vi "Store Reference.vi"(8 "error in":errorcluster, 11 "Reference":variant) -> (0 "error out":errorcluster, 3 "id":string)   [LabVIEW 2020, in "G-AI Core.lvlib"]
doc: "Stores a reference (e.g. VI Reference, Control Reference ...) in the G-AI Core and returns a unique id for later use of that reference.\n\n_____\nCreated using DQMH Framework: Event Scripter 7.1.2.1547."
uses:
  G-AI Core.lvlib
  Store Reference Argument--cluster.ctl
  Store Reference (Reply Payload)--cluster.ctl
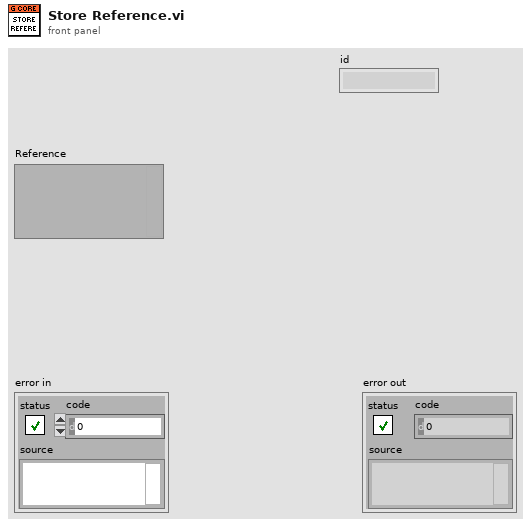
[diagram p1: front panel]
types:
  T1 = typedef "G-AI Core.lvlib/Store Reference Argument--cluster.ctl" = cluster{"Reference":variant, "Wait Notifier":refnum<notifier>, "wait for reply":bool}
  T2 = typedef "G-AI Core.lvlib/Request Events--cluster.ctl" = cluster{"Stop Module":refnum<user-event>, "Show Panel":refnum<user-event>, "Hide Panel":refnum<user-event>, "Get Module Execution Status":refnum<user-event>, "Show Diagram":refnum<user-event>, "Store Reference":refnum<user-event>, "Get Reference":refnum<user-event>, "New VI":refnum<user-event>, "Open VI Reference":refnum<user-event>}
  T3 = typedef "G-AI Core.lvlib/Store Reference (Reply Payload)--cluster.ctl" = cluster{"id":string, "error":errorcluster}
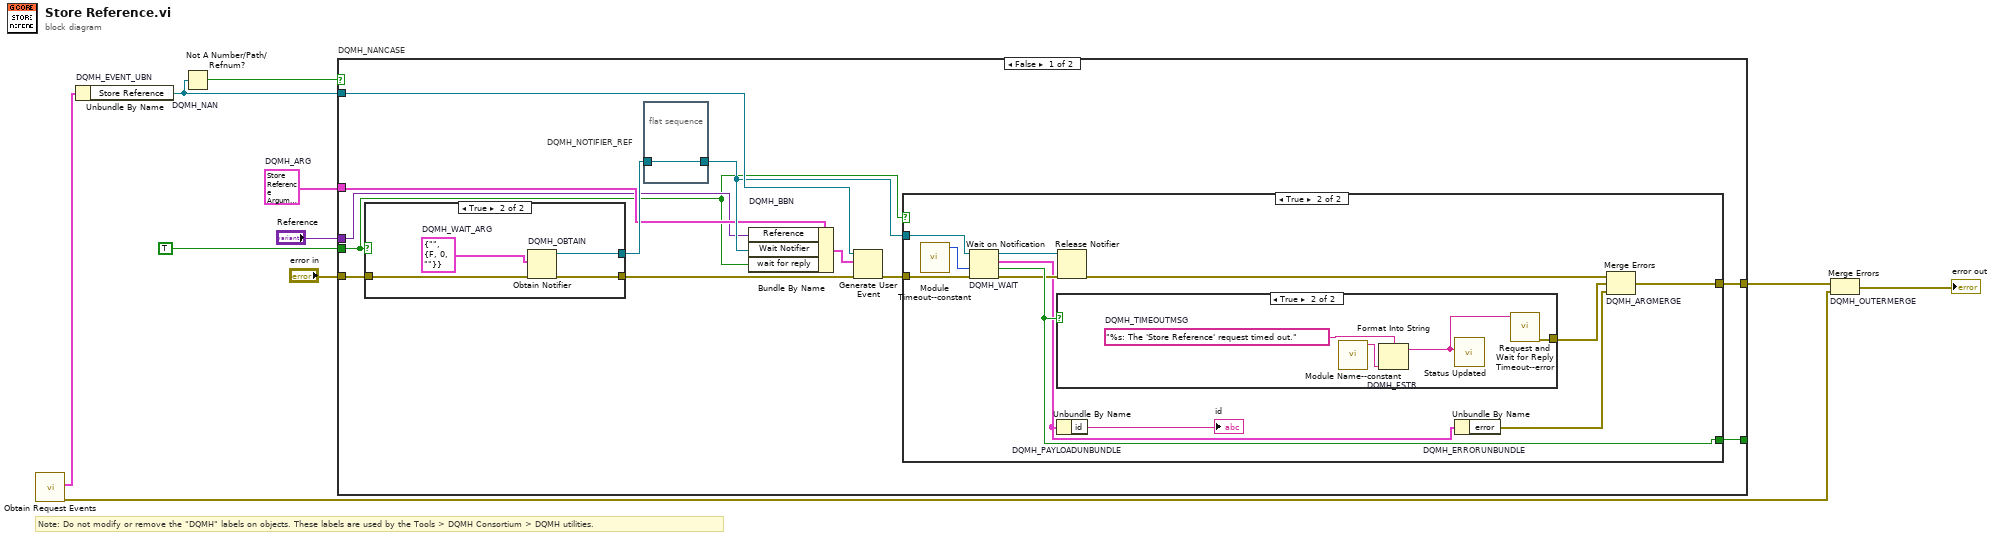
[diagram p0: block diagram]
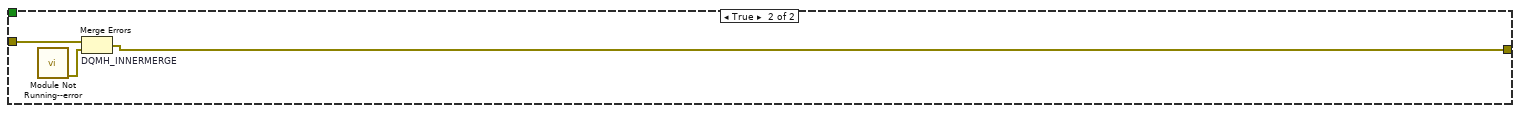
[diagram p5: hidden frame]
diagram:
  w5 = T1 {"Reference"=variant, "Wait Notifier"=refnum, "wait for reply"=FALSE}  # DQMH_ARG
  # "Note: Do not modify or remove the \"DQMH\" labels on objects. These labels are used by the Tools > DQMH Consortium > DQMH utilities."
  n1 = call "Obtain Request Events.vi"() -> ("error out"=w2:errorcluster, "G-AI Core Request Events"=w1:T2)  [unwired: 10 in]
  n2 = Unbundle By Name "DQMH_EVENT_UBN"(w1) -> ("Store Reference"=w8:refnum<user-event>)
  n3 = Not A Number/Path/Refnum? "DQMH_NAN"(number/path/refnum=w8) -> (NaN/Path/Refnum?=w7:bool)
  n4 = case "DQMH_NANCASE" shown="False" w7 {
    tunnel: "error in" -> [w22 w48]
    tunnel: w8 -> [w20 _]
    tunnel: [w17 w47] -> w6
    tunnel: [w18 _] -> _
    tunnel: w5 -> [w13 _]
    tunnel: "Reference" -> [w12 _]
    tunnel: TRUE ("wait for reply (T)") -> [w11 _]
    frame False {
      n5 = case shown="True" w11 {
        tunnel: w22 -> [w41 w45]
        tunnel: [w41 w44] -> w19
        tunnel: [_ w42] -> w15
        frame False {
        }
        frame True {
          w43 = T3 {"id"="", "error"={"status"=FALSE, "code"=0, "source"=""}}  # DQMH_WAIT_ARG
          n6 = Obtain Notifier "DQMH_OBTAIN"(notification data type=w43, error in (no error)=w45) -> (notifier out=w42:refnum<notifier>, error out=w44:errorcluster)  [unwired: 2 in, 1 out]
        }
      }
      n7 = flat-sequence "DQMH_NOTIFIER_REF" {
        tunnel: w15 -> [w23]
        tunnel: [w23] -> w14
        frame #0 {
        }
      }
      n8 = Bundle By Name "DQMH_BBN"(cluster=w13, "Reference"=w12, "Wait Notifier"=w14, "wait for reply"=w11) -> (w16:T1)
      n9 = Generate User Event(user event=w20, event data cluster=w16, error in=w19) -> (error out=w21:errorcluster)  [unwired: 1 in, 1 out]
      n10 = case shown="True" w11 {
        tunnel: w21 -> [w24 w36]
        tunnel: w14 -> [_ w35]
        tunnel: [_ w33] -> w18
        tunnel: [w24 w32] -> w17
        frame False {
        }
        frame True {
          n11 = call "Module Timeout--constant.vi"() -> ("Module Timeout"=w26:i32)  [unwired: 11 in]
          n12 = Wait on Notification "DQMH_WAIT"(notifier=w35, timeout in ms (-1)=w26, error in (no error)=w36) -> (notifier out=w34:refnum<notifier>, notification=w27:T3, timed out?=w33:bool, error out=w31:errorcluster)  [unwired: 1 in]
          n13 = case shown="True" w33 {
            tunnel: [_ w38] -> w28
            frame False {
            }
            frame True {
              w40 = "%s: The 'Store Reference' request timed out."  # DQMH_TIMEOUTMSG
              n14 = call "Module Name--constant.vi"() -> ("Module Name"=w37:string)  [unwired: 11 in]
              n15 = Format Into String "DQMH_FSTR"(format string=w40, w37) -> (resulting string=w39:string)  [unwired: 2 in, 1 out]
              n16 = call "Status Updated.vi"("Status"=w39) -> ()  [unwired: 10 in, 1 out]
              n17 = call "Request and Wait for Reply Timeout--error.vi"("Error Message"=w39) -> ("error out"=w38:errorcluster)  [unwired: 10 in]
            }
          }
          n18 = Unbundle By Name "DQMH_PAYLOADUNBUNDLE"(w27) -> ("id"=→"id":string)
          n19 = Release Notifier(notifier=w34, error in (no error)=w31) -> (error out=w30:errorcluster)  [unwired: 1 in, 2 out]
          n20 = Unbundle By Name "DQMH_ERRORUNBUNDLE"(w27) -> ("error"=w29:errorcluster)
          n21 = Merge Errors "DQMH_ARGMERGE"(w30, w28, w29) -> (w32:errorcluster)
        }
      }
    }
    frame True {
      n22 = call "Module Not Running--error.vi"() -> ("error out"=w46:errorcluster)  [unwired: 11 in]
      n23 = Merge Errors "DQMH_INNERMERGE"(w48, w46) -> (w47:errorcluster)
    }
  }
  n24 = Merge Errors "DQMH_OUTERMERGE"(w6, w2) -> (→"error out":errorcluster)
